vi "Set Table Record.vi"(1 "Data In":T1) -> (0 "Record Out":string[](array[string]))   [LabVIEW 2018]
uses:
  Ctls/DisplayIndicator.ctl
  Ctls/MotroConfigData.ctl
  Ctls/MotorConfig.ctl
  Ctls/MagType.ctl
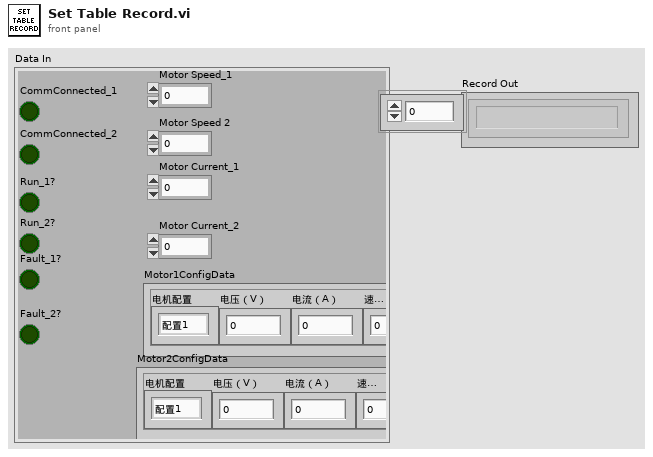
[diagram p1: front panel]
types:
  T1 = typedef "DisplayIndicator.ctl" = cluster{"CommConnected_1":bool, "Run_1?":bool, "Fault_1?":bool, "CommConnected_2":bool, "Run_2?":bool, "Fault_2?":bool, "Motor Speed 2":sgl, "Motor Speed_1":sgl, "Motor Current_1":sgl, "Motor Current_2":sgl, "Motor1ConfigData":T2, "Motor2ConfigData":T2}
  T2 = typedef "MotroConfigData.ctl" = cluster{"电机配置":T3, "电压（V）":dbl, "电流（A）":dbl, "速度（RPM）":dbl, "励磁方式":T4}
  T3 = typedef "MotorConfig.ctl" = enum16{"配置1", "配置2", "配置3", "配置4"}
  T4 = typedef "MagType.ctl" = enum16{"永磁", "励磁"}
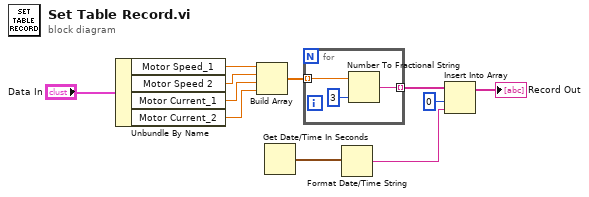
[diagram p0: block diagram]
diagram:
  n1 = Unbundle By Name("Data In") -> ("Motor Speed_1"=w5:sgl, "Motor Speed 2"=w6:sgl, "Motor Current_1"=w7:sgl, "Motor Current_2"=w8:sgl)
  n2 = Build Array(w5, w6, w7, w8) -> (w9:sgl[])
  n3 = Get Date/Time In Seconds() -> (seconds since 1Jan1904=w2:timestamp)
  n4 = for {
    tunnel: w9 -> [w13] mode=indexing
    tunnel: [w12] -> w10 mode=indexing
    n5 = Number To Fractional String(number=w13, precision (6)=i16 3) -> (F-format string=w12:string)  [unwired: 2 in]
  }
  n6 = Format Date/Time String(seconds (now)=w2) -> (date/time string=w1:string)  [unwired: 2 in]
  n7 = Insert Into Array(array=w10, index=0, new element=w1) -> (→"Record Out":string[])
